vi "Calibrate Arm.vi"(8 "error in (no error)":errorcluster, 11 "KUKA youBot arm_EtherCAT in":refnum<class "NI_Robotics_KUKA youBot Arm_EtherCAT.lvclass">) -> (0 "error out":errorcluster, 3 "KUKA youBot arm_EtherCAT out":refnum<class "NI_Robotics_KUKA youBot Arm_EtherCAT.lvclass">)   [LabVIEW 2017, in "NI_Robotics_KUKA youBot Host.lvlib" / "NI_Robotics_KUKA youBot Arm_EtherCAT.lvclass"]
uses:
  <vilib>/robotics/KUKA youBot/Basic Device/Arm EtherCAT/NI_Robotics_KUKA youBot Arm_EtherCAT.lvclass
  c:/Program Files (x86)/National Instruments/LabVIEW 2017/vi.lib/robotics/KUKA youBot/Basic Device/Arm/NI_Robotics_KUKA youBot Arm.lvclass
  <vilib>/robotics/KUKA youBot/Motor/Arm Motor/NI_Robotics_KUKA youBot Arm Motor.lvclass
  <vilib>/robotics/KUKA youBot/Basic Device/Arm/NI_Robotics_KUKA youBot Arm.lvclass
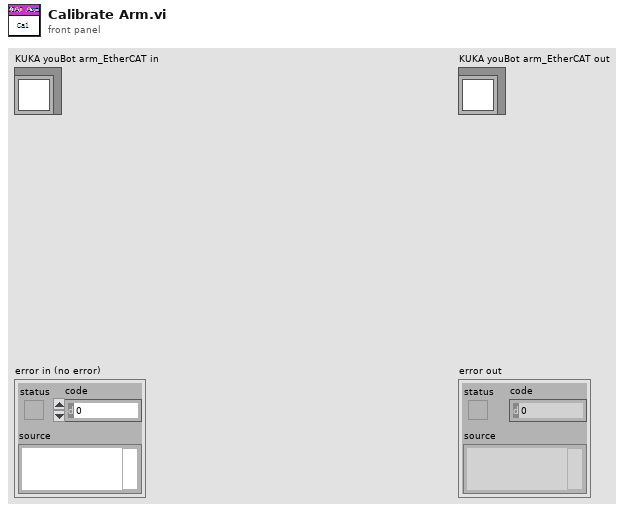
[diagram p1: front panel]
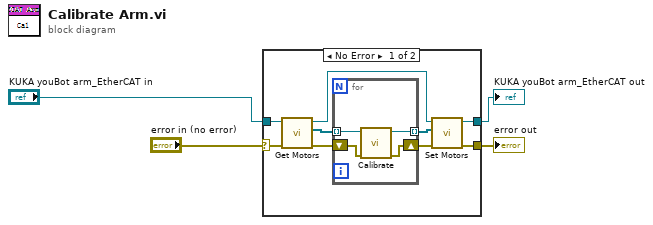
[diagram p0: block diagram]
diagram:
  n1 = case shown="No Error" "error in (no error)" {
    selector: "error in (no error)" -> [w12 w18]
    tunnel: "KUKA youBot arm_EtherCAT in" -> [w13 w19]
    tunnel: [w6 w18] -> w2
    tunnel: [w5 w19] -> w1
    frame No Error {
      n2 = call-dynamic "Get Motors.vi"("error in (no error)"=w12, "KUKA youBot arm in"=w13) -> ("error out"=w10:errorcluster, "motors"=w11:refnum<class "NI_Robotics_KUKA youBot Arm Motor.lvclass">[], "KUKA youBot arm out"=w8:refnum<class "NI_Robotics_KUKA youBot Arm_EtherCAT.lvclass">)  [unwired: 7 in]
      n3 = for {
        tunnel: w11 -> [w17] mode=indexing
        shift-right: [w15] -> w9
        shift-left: w10 -> [w16]
        tunnel: [w14] -> w7 mode=indexing
        n4 = call-dynamic "Calibrate.vi"("error in (no error)"=w16, "KUKA youBot arm motor in"=w17) -> ("error out"=w15:errorcluster, "KUKA youBot arm motor out"=w14:refnum<class "NI_Robotics_KUKA youBot Arm Motor.lvclass">)  [unwired: 8 in]
      }
      n5 = call <vilib>:"Set Motors.vi"("error in (no error)"=w9, "motors"=w7, "KUKA youBot arm in"=w8) -> ("error out"=w6:errorcluster, "KUKA youBot arm out"=w5:refnum<class "NI_Robotics_KUKA youBot Arm_EtherCAT.lvclass">)  [unwired: 7 in]
    }
    frame Error {
    }
  }
  "error out" <- w2
  "KUKA youBot arm_EtherCAT out" <- w1
